vi "PicoScope2000GetStreamingValues.vi"(10 "handle in":i16, 11 "error in":errorcluster) -> (0 "App Buffer startIndex":u32, 1 "Trigger":cluster{bool, "triggeredAt  Index (Total)":u32}, 2 "handle out":i16, 3 "error out":errorcluster, 4 "Number of Samples":u32, 5 "ready":i16, 6 "Auto Stopped":bool, 7 "Application Buffer Full":bool, 8 "overflow":i16 format="%02b", 9 "Total Samples":u32)   [LabVIEW 2010]
doc: "This VI is used in streaming mode to get the latest values from the driver. It should be called in a loop after the oscilloscope has been set up using PicoScope3000aSettings.vi and streaming has been started by calling PicoScope3000aStartStreaming.vi. The VI outputs the number of samples available and the start index of these samples in the array output by PicoScope3000aStartStreaming.vi."
uses:
  ps2000Wrap.dll
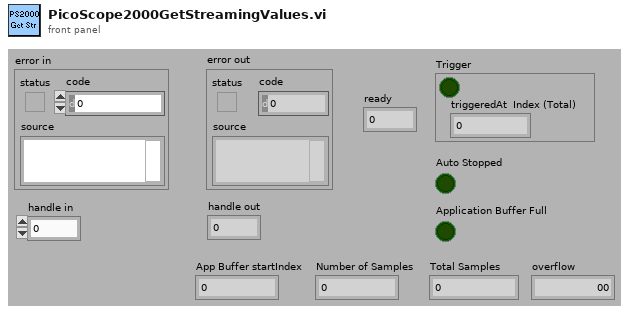
[diagram p1: front panel]
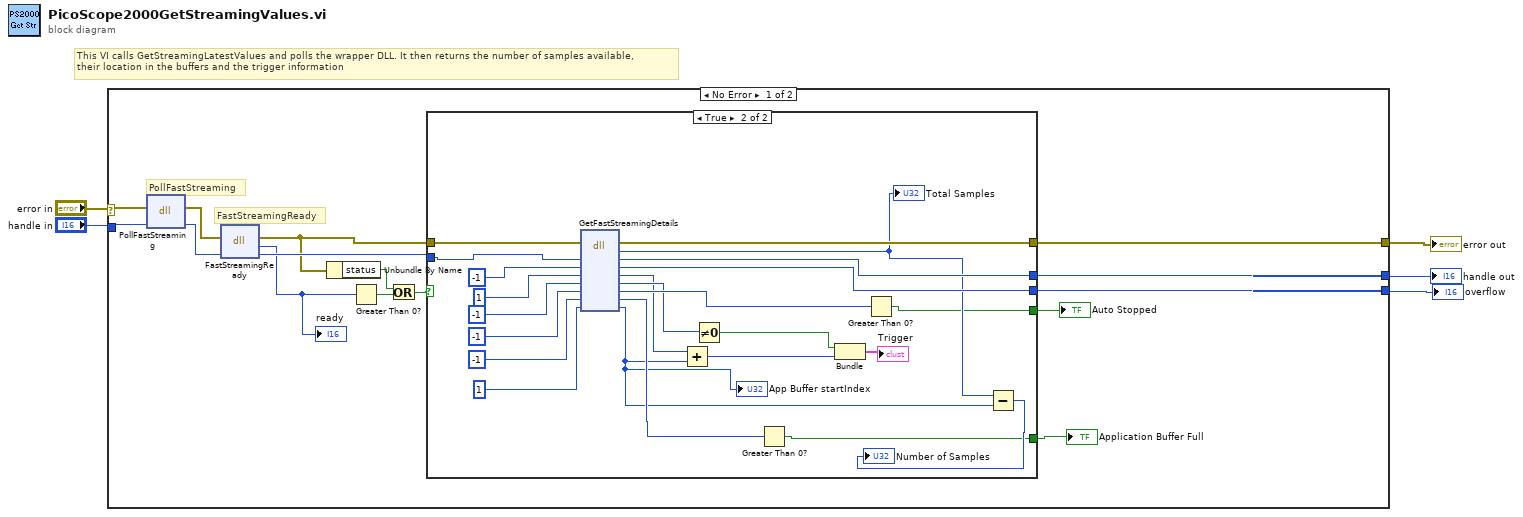
[diagram p0: block diagram]
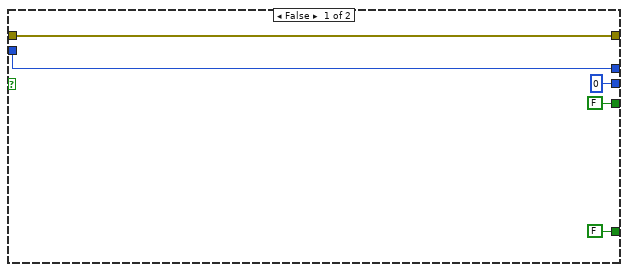
[diagram p2: hidden frame]
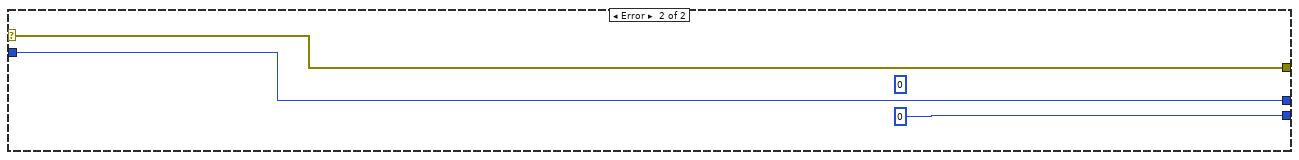
[diagram p3: hidden frame]
diagram:
  # "This VI calls GetStreamingLatestValues and polls the wrapper DLL. It then returns the number of samples available, \ntheir location in the buffers and the trigger information"
  n1 = case shown="No Error" "error in" {
    selector: "error in" -> [w6 w51]
    tunnel: [w20 w51] -> w4
    tunnel: "handle in" -> [w7 w50]
    tunnel: [w19 w50] -> w2
    tunnel: [w11 i16 0 ("overflow")] -> w1
    frame No Error {
      # "PollFastStreaming"
      # "FastStreamingReady"
      n2 = dll-call lib="ps2000Wrap.dll" fn="PollFastStreaming" ("PS5000.dll:_ps5000SetDataBuffer@16")(error in=w6, "handle"=w7) -> (error out=w14:errorcluster, "handle"=w15:i16)  [unwired: 3 in, 1 out]
      n3 = dll-call lib="ps2000Wrap.dll" fn="FastStreamingReady" ("PS5000.dll:_ps5000SetDataBuffer@16")(error in=w14, "handle"=w15) -> (error out=w10:errorcluster, "ready"=w12:i16, "handle"=w13:i16)  [unwired: 2 in, 1 out]
      "ready" <- w12
      n4 = Unbundle By Name(w10) -> ("status"=w17:bool)
      n5 = Greater Than 0?(x=w12) -> (x > 0?=w18:bool)
      n6 = Or(x=w17, y=w18) -> (x .or. y?=w16:bool)
      n7 = case shown="True" w16 {
        tunnel: [w25 w39] -> w20
        tunnel: w13 -> [w24 w40]
        tunnel: w10 -> [w25 w41]
        tunnel: [w24 w38] -> w19
        tunnel: [i16 0 ("overflow") w37] -> w11
        tunnel: [FALSE w33] -> w9
        tunnel: [FALSE w32] -> w8
        frame False {
        }
        frame True {
          n8 = dll-call lib="ps2000Wrap.dll" fn="GetFastStreamingDetails"(error in=w41, "handle"=w40, "overflow"=i16 -1, "triggeredAt"=u32 1, "triggered"=i16 -1, "auto_stop"=i16 -1, "appBufferFull"=i16 -1, "startIndex"=u32 1) -> (error out=w39:errorcluster, "totalValues"=w34:u32, "handle"=w38:i16, "overflow"=w37:i16, "triggeredAt"=w45:u32, "triggered"=w47:i16, "auto_stop"=w48:i16, "appBufferFull"=w46:i16, "startIndex"=w35:u32)  [unwired: 2 in, 1 out]
          "App Buffer startIndex" <- w35
          "Total Samples" <- w34
          n9 = Add(x=w45, y=w35) -> (x+y=w42:u32)
          n10 = Not Equal To 0?(x=w47) -> (x != 0?=w43:bool)
          n11 = Greater Than 0?(x=w46) -> (x > 0?=w32:bool)
          n12 = Bundle(w43, w42) -> (→"Trigger":cluster{bool, u32})  [unwired: 1 in]
          n13 = Greater Than 0?(x=w48) -> (x > 0?=w33:bool)
          n14 = Subtract(x=w34, y=w35) -> (x-y=→"Number of Samples":u32)
        }
      }
      "Auto Stopped" <- w9
      "Application Buffer Full" <- w8
    }
    frame Error {
      (unwired) u32 0 ("totalValues")
    }
  }
  "error out" <- w4
  "handle out" <- w2
  "overflow" <- w1
